vi "mainBackup.vi"() -> ()   [LabVIEW 2013]
uses:
  DB/ConfEnum.ctl
  DB/DbEnum.ctl
  DB/ConfDB.ctl
panel:
  in  "File Name 2":string
  in  "Path":path
  out "XY Graph":cluster{u32[], i32[]}(graph)
  in  "Start Index 2":i32
  in  "error in 2":errorcluster
  out "Image Out":T1(plugin-control)
  in  "N times sigam (tol)":i32
  in  "Number of images to save around freeze point":i32
  in  "Number of Images":i32
  in  "File Path":path
  out "Number of Matches":i32
  out "Matches (pixel)":T2(array[cluster])
  in  "File Name":string
  in  "Start Index":i32
  out "error out":errorcluster
  in  "error in":errorcluster
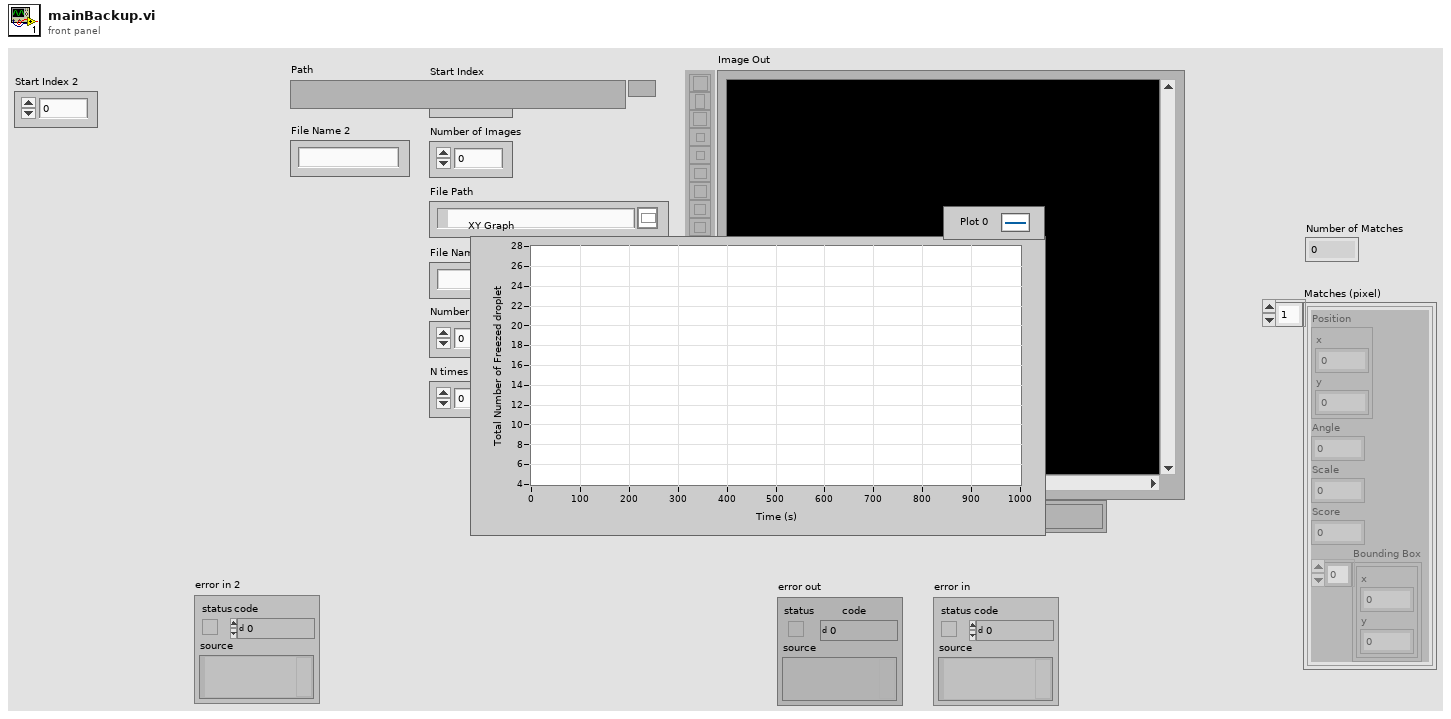
[diagram p1: front panel]
types:
  T1 = typedef "IMAQ Image.ctl" = refnum<image>
  T2 = cluster{"Position":cluster{"x":sgl, "y":sgl}, "Angle":sgl, "Scale":sgl, "Score":sgl, "Bounding Box":cluster{"x":sgl, "y":sgl}[]}[]
  T3 = typedef "ConfDB.ctl" = cluster{"NumberOfImages":i32, "NoImages2SaveAroundFreeze":i32, "Path":path, "NameOfPartialFile":string, "StartIndex":i32, "NumberOfStdTol":i32}
  T4 = typedef "DbEnum.ctl" = enum16{"Init", "Insert Detection Result Data", "GetDropletsBoundingBox"}
  T5 = typedef "ConfEnum.ctl" = enum16{"Init", "GetFileNameStartIndex", "Configure DB"}
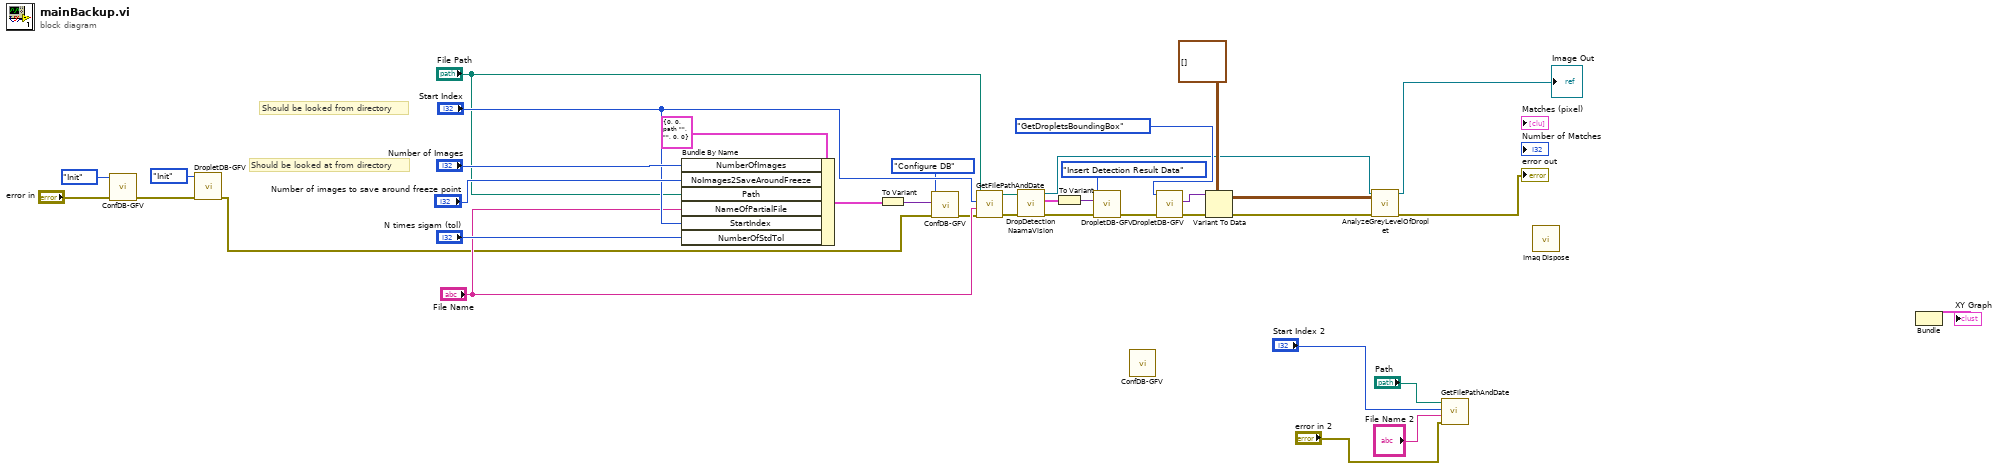
[diagram p0: block diagram]
diagram:
  # "Should be looked from directory"
  # "Should be looked at from directory"
  n1 = call "ConfDB-GFV.vi"("error in (no error)"="error in", "Command In"=ConfEnum."Init" ("Command")) -> ("error out"=w21:errorcluster)  [unwired: 8 in, 1 out]
  n2 = call "DropletDB-GFV.vi"("error in (no error)"=w21, "Command In"=DbEnum."Init") -> ("error out"=w28:errorcluster)  [unwired: 8 in, 1 out]
  n3 = Bundle By Name(cluster=T3 {"NumberOfImages"=0, "NoImages2SaveAroundFreeze"=0, "Path"=path "", "NameOfPartialFile"="", "StartIndex"=0, "NumberOfStdTol"=0} ("ConfDB"), "NumberOfImages"="Number of Images", "NoImages2SaveAroundFreeze"="Number of images to save around freeze point", "Path"="File Path", "NameOfPartialFile"="File Name", "StartIndex"="Start Index", "NumberOfStdTol"="N times sigam (tol)") -> (w33:T3)
  n4 = To Variant(anything=w33) -> (Variant=w32:variant)
  n5 = call "ConfDB-GFV.vi"("error in (no error)"=w28, "Data in"=w32, "Command In"=ConfEnum."Configure DB") -> ("error out"=w31:errorcluster)  [unwired: 7 in, 1 out]
  n6 = call "GetFilePathAndDate.vi"("error in (no error)"=w31, "String"="File Name", "Index"="Start Index", "Path"="File Path") -> ("error out"=w24:errorcluster, "file out"=w40:path)  [unwired: 5 in, 1 out]
  n7 = call "DropDetection NaamaVision.vi"("error in"=w24, "Path"=w40) -> ("error out"=w23:errorcluster, "Matches (pixel)"=w27:T2, "Image Out"=w12:T1)  [unwired: 6 in, 1 out]
  n8 = To Variant(anything=w27) -> (Variant=w26:variant)
  n9 = call "DropletDB-GFV.vi"("error in (no error)"=w23, "Data in"=w26, "Command In"=DbEnum."Insert Detection Result Data") -> ("error out"=w18:errorcluster)  [unwired: 7 in, 1 out]
  n10 = call "ConfDB-GFV.vi"() -> ()  [unwired: 10 in, 2 out]
  n11 = call "DropletDB-GFV.vi"("error in (no error)"=w18, "Command In"=DbEnum."GetDropletsBoundingBox") -> ("error out"=w16:errorcluster, "Data out"=w15:variant)  [unwired: 8 in]
  n12 = Variant To Data(error in=w16, type=cluster{"x":sgl, "y":sgl}[][] [] ("Bounding Box"), Variant=w15) -> (data=w13:cluster{"x":sgl, "y":sgl}[][], error out=w11:errorcluster)
  n13 = call "AnalyzeGreyLevelOfDroplet.vi"("error in (no error)"=w11, "Bounding Box"=w13, "Image In"=w12) -> ("error out"=→"error out":errorcluster, "Image Out"=→"Image Out":T1)  [unwired: 6 in, 1 out]
  n14 = call "GetFilePathAndDate.vi"("error in (no error)"="error in 2", "String"="File Name 2", "Index"="Start Index 2", "Path"="Path") -> ("error out"=w5:errorcluster, "creation date"=w1:u32, "file out"=w4:path)  [unwired: 5 in]
  n15 = call "Imaq Dispose"() -> ()  [unwired: 6 in, 1 out]
  n16 = Bundle() -> (→"XY Graph":cluster{void, void})  [unwired: 3 in]
